vi "Oneshot Tester.vi"() -> ()   [LabVIEW 2024]
uses:
  definitions/volume.type--enum.ctl
panel:
  out "current volume":string
  out "Array":string[](array[string])
  in  "Folder Path":path=path "D:/Comics/data/cv_volumes"
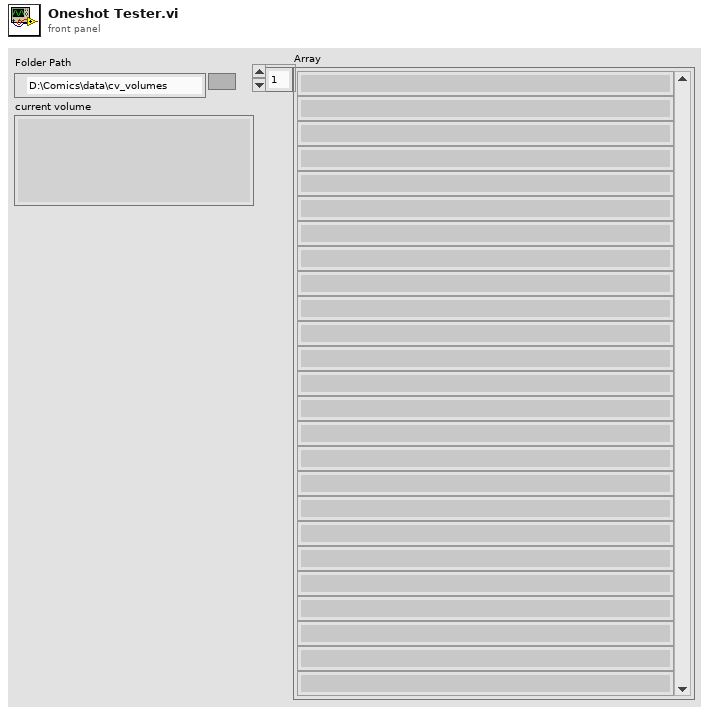
[diagram p1: front panel]
types:
  T1 = typedef "volume.type--enum.ctl" = enum16{"Ongoing", "Limited Series", "Annual", "One Shot", "Reprint/Document"}
  T2 = typedef "local_volume.ctl" = cluster{"id":i32, "name":string, "sortable_name":string, "aliases":string[], "description":string, "site_detail_url":string, "count_of_issues":i32, "start_year":i32, "publisher_id":i32, "issue_ids":i32[], "date_last_updated":timestamp, "volume":i32, "cv_id":string, "volume type":T1}
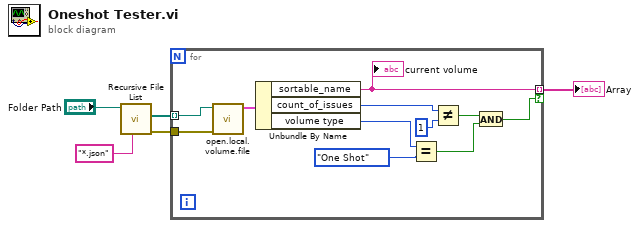
[diagram p0: block diagram]
diagram:
  n1 = call <vilib>:"Recursive File List.vi"("pattern"="*.json", "Folder Path"="Folder Path") -> ("error out"=w3:errorcluster, "All Files in Dir"=w2:path[])  [unwired: 5 in, 3 out]
  n2 = for {
    tunnel: w3 -> [w16]
    tunnel: w2 -> [w15] mode=indexing
    tunnel: [w9] -> w1 mode=indexing if=w6
    n3 = call "open.local.volume.file.vi"("error in (no error)"=w16, "volume json"=w15) -> ("volume"=w14:T2)  [unwired: 8 in, 1 out]
    n4 = Unbundle By Name(w14) -> ("sortable_name"=w9:string, "count_of_issues"=w11:i32, "volume type"=w13:T1)
    "current volume" <- w9
    n5 = Equal?(x=w13, y=volume.type--enum."One Shot") -> (x = y?=w7:bool)
    n6 = Not Equal?(x=w11, y=1) -> (x != y?=w8:bool)
    n7 = And(x=w8, y=w7) -> (x .and. y?=w6:bool)
  }
  "Array" <- w1
